vi "Set Laser PWM.vi"(8 "error in (no error)":errorcluster, 10 "PWM Duty cycle":u8, 11 "VISA Refnum in":refnum<visa-resource-name>) -> (0 "error out":errorcluster, 3 "VISA Refnum out":refnum<visa-resource-name>)   [LabVIEW 2020, in "Control de MaP.lvlib"]
uses:
  Control de MaP.lvlib
  Write--command.vi
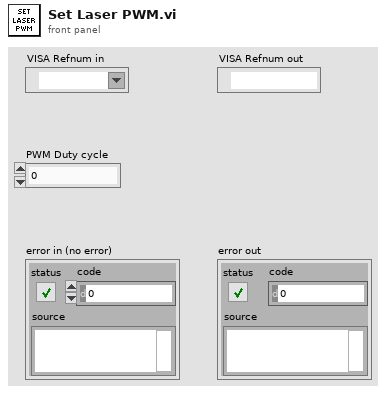
[diagram p1: front panel]
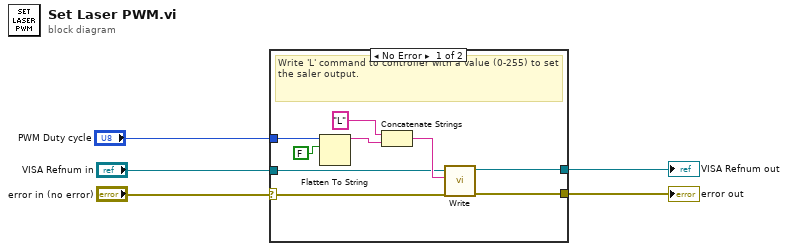
[diagram p0: block diagram]
diagram:
  n1 = case shown="No Error" "error in (no error)" {
    selector: "error in (no error)" -> [w7 w15]
    tunnel: "PWM Duty cycle" -> [w11 _]
    tunnel: [w10 w16] -> w4
    tunnel: "VISA Refnum in" -> [w9 w16]
    tunnel: [w8 w15] -> w2
    frame No Error {
      # "Write 'L' command to controller with a value (0-255) to set the saler output."
      n2 = Flatten To String(anything=w11, prepend array or string size? (T)=FALSE) -> (data string=w13:string)  [unwired: 2 in, 2 out]
      n3 = Concatenate Strings("L" ("Command"), w13) -> (w14:string)
      n4 = call-poly "Write.vi"("error in (no error)"=w7, "Command"=w14, "VISA resource name"=w9) -> ("error out"=w8:errorcluster, "VISA resource name out"=w10:refnum<visa-resource-name>)  [unwired: 6 in, 1 out]
    }
    frame Error {
    }
  }
  "VISA Refnum out" <- w4
  "error out" <- w2
